vi "Main.vi"(8 "error in (no error)":errorcluster, 11 "UIEvents":refnum<user-event>) -> (0 "error out":errorcluster)   [LabVIEW 2020, in "SensorInterface.lvlib"]
doc: "Use this template to build a producer/consumer design pattern with events to produce queue items. Use this design pattern instead of the User Interface Event Handler pattern for user interfaces when you want to execute code asynchronously in response to an event without slowing the user interface responsiveness."
uses:
  SensorInterface.lvlib
  Controls/QMessage.ctl
  Support/UserEvents/Controls/EventMessage.ctl
  Controls/ConsummerLoopData.ctl
  Controls/EventLoopData.ctl
panel:
  out "ModuleQ Out":refnum<queue>
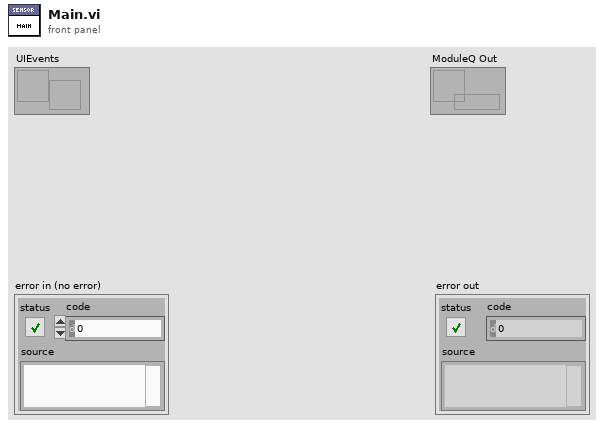
[diagram p1: front panel]
types:
  T1 = typedef "SensorInterface.lvlib/EventLoopData.ctl" = cluster{"DummyData":dbl}
  T2 = typedef "SensorInterface.lvlib/ConsummerLoopData.ctl" = cluster{"Error File Refnum":refnum<file>}
  T3 = typedef "Template.lvlib/QMessage.ctl" = cluster{"Command":string, "Data":variant}
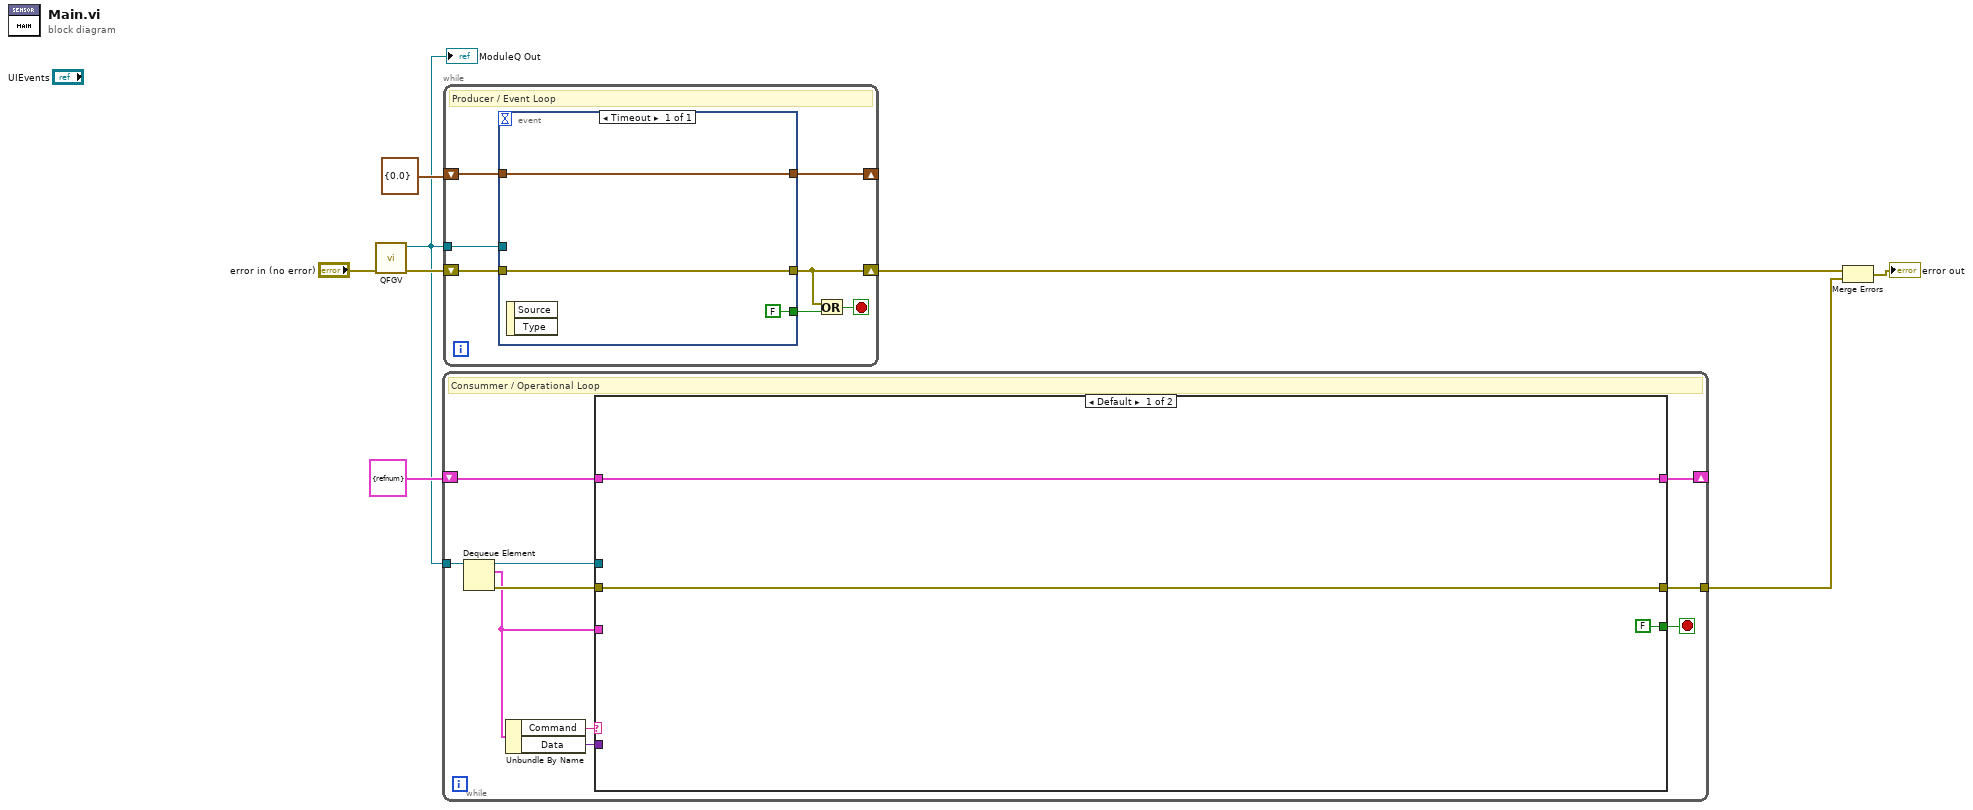
[diagram p0: block diagram]
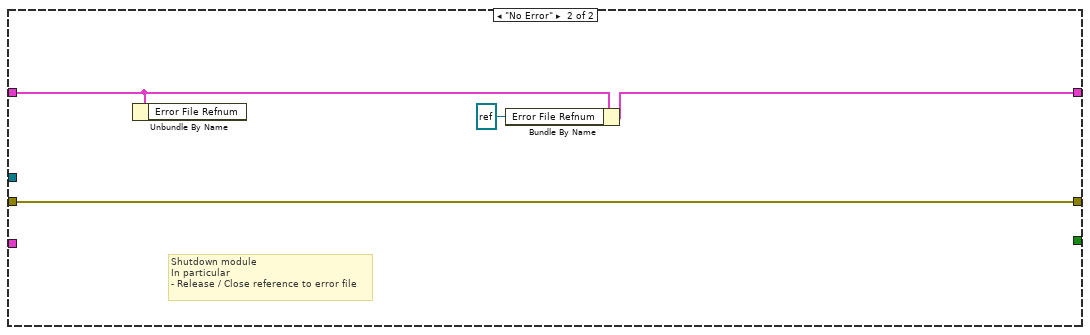
[diagram p2: hidden frame]
diagram:
  n1 = call "QFGV.vi"("error in (no error)"="error in (no error)") -> ("error out"=w2:errorcluster, "ModuleQ"=w1:refnum<queue>)  [unwired: 9 in]
  "ModuleQ Out" <- w1
  n2 = while {
    tunnel: w1 -> [w18]
    shift-right: [w16] -> _
    shift-left: T2 {"Error File Refnum"=refnum} -> [w15]
    tunnel: [w13] -> w7
    stop <- w17 stop-if-true
    # "Consummer / Operational Loop"
    n3 = Dequeue Element(queue=w18) -> (queue out=w12:refnum<queue>, element=w11:T3, error out=w14:errorcluster)  [unwired: 2 in, 1 out]
    n4 = Unbundle By Name(w11) -> ("Command"=w10:string, "Data"=w9:variant)
    n5 = case shown="Default" w10 {
      tunnel: [FALSE _] -> w17
      tunnel: [w20 w23] -> w16
      tunnel: w15 -> [w20 w24]
      tunnel: w14 -> [w19 w25]
      tunnel: [w19 w25] -> w13
      tunnel: w12 -> [_ _]
      tunnel: w11 -> [_ _]
      tunnel: w9 -> [_ _]
      frame Default {
      }
      frame "No Error" {
        # "Shutdown module\nIn particular\n- Release / Close reference to error file"
        n6 = Unbundle By Name(w24) -> ()  [unwired: 1 out]
        n7 = Bundle By Name(cluster=w24, "Error File Refnum"=refnum<file> refnum) -> (w23:T2)
      }
    }
  }
  n8 = while {
    shift-right: [w28] -> w6
    shift-left: w2 -> [w31]
    tunnel: w1 -> [w32]
    shift-right: [w27] -> _
    shift-left: T1 {"DummyData"=0.0} -> [w26]
    stop <- w29 stop-if-true
    # "Producer / Event Loop"
    n9 = event shown="[0] Timeout" {
      selector: _ -> [_]
      dyn-events: _ -> [_]
      timeout: _ -> [_]
      tunnel: w32 -> [_]
      tunnel: w31 -> [w34]
      tunnel: [w34] -> w28
      tunnel: [FALSE ("stop")] -> w30
      tunnel: [w35] -> w27
      tunnel: w26 -> [w35]
      event Timeout {
        n10 = event-data() -> ()  [unwired: 1 in, 2 out]
      }
    }
    n11 = Or(x=w28, y=w30) -> (x .or. y?=w29:bool)
  }
  n12 = Merge Errors(w6, w7) -> (→"error out":errorcluster)
